vi "Calibration Cal IsNeeded Set InstDriver Handle in.vi"(8 "error in (no error)":errorcluster, 10 "InstDriver Handle in":T1, 11 "niDTS Calibration Cal IsNeeded RF Test in":refnum<class "niDTS Calibration Cal IsNeeded RF Test.lvclass">) -> (0 "error out":errorcluster, 3 "niDTS Calibration Cal IsNeeded RF Test out":refnum<class "niDTS Calibration Cal IsNeeded RF Test.lvclass">)   [LabVIEW 2015, in "niDTS Utilities.lvlib" / "niDTS Calibration Cal IsNeeded RF Test.lvclass"]
uses:
  niDTS Calibration Cal IsNeeded RF Test.lvclass
  RiviInstDriver/niRfGeneralSettings/Includes/niRfGeneralSettings INC Handle.ctl
  RiviInstDriver/niRfGeneralSettings/Objects/niRfGeneralSettings.lvclass
  niDTS Calibration Cal IsNeeded RF Test.lvclass/niDTS Calibration Cal IsNeeded RF Test.ctl
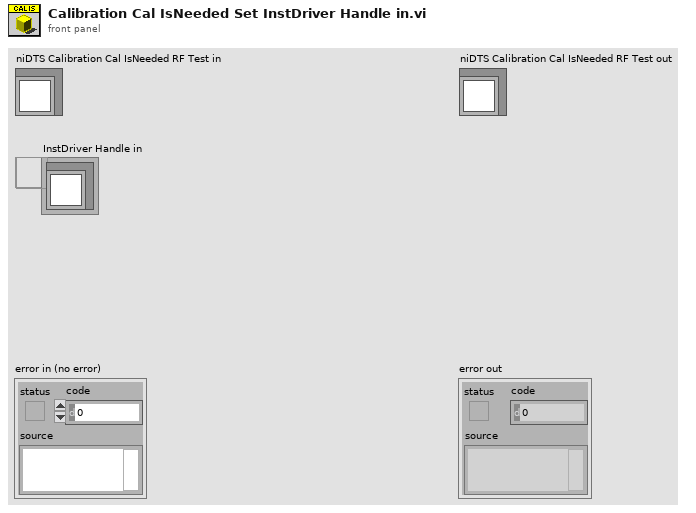
[diagram p1: front panel]
types:
  T1 = typedef "niRfGeneralSettings.lvclass/niRfGeneralSettings INC Handle.ctl" = refnum<data-value>
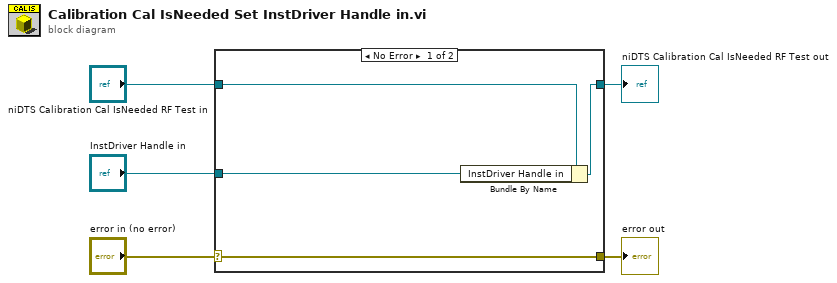
[diagram p0: block diagram]
diagram:
  n1 = case shown="No Error" "error in (no error)" {
    selector: "error in (no error)" -> [w9 w10]
    tunnel: [w9 w10] -> w4
    tunnel: [w7 w11] -> w2
    tunnel: "niDTS Calibration Cal IsNeeded RF Test in" -> [w8 w11]
    tunnel: "InstDriver Handle in" -> [w6 _]
    frame No Error {
      n2 = Bundle By Name(cluster=w8, "InstDriver Handle in"=w6) -> (w7:refnum<class "niDTS Calibration Cal IsNeeded RF Test.lvclass">)
    }
    frame Error {
    }
  }
  "error out" <- w4
  "niDTS Calibration Cal IsNeeded RF Test out" <- w2
